vi "DO_init.vi"(0 "DOParameters":string[](array[string]), 1 "N_param":i32, 2 "N_moduls":i32, 5 "Parameters def":i32[][](array[numeric]), 7 "Names def":string[][](array[string]), 9 "KFM":string[](array[string]), 12 "conninfo":T1={"host"="localhost", "port"="5432", "client_encoding"="WIN1251", "dbname"="data", "user"="postgres", "password"=""}, 13 "DOParamTable":string="fdo_3") -> (4 "DO out":T2, 15 "error":errorcluster)   [LabVIEW 2019, in "Inputs.lvlib"]
uses:
  Inputs.lvlib
  Ctl/DO.ctl
  Ctl/Parameter State.ctl
  Database/ctl/Coninfo.ctl
  Database/PostgreSQL.lvlib
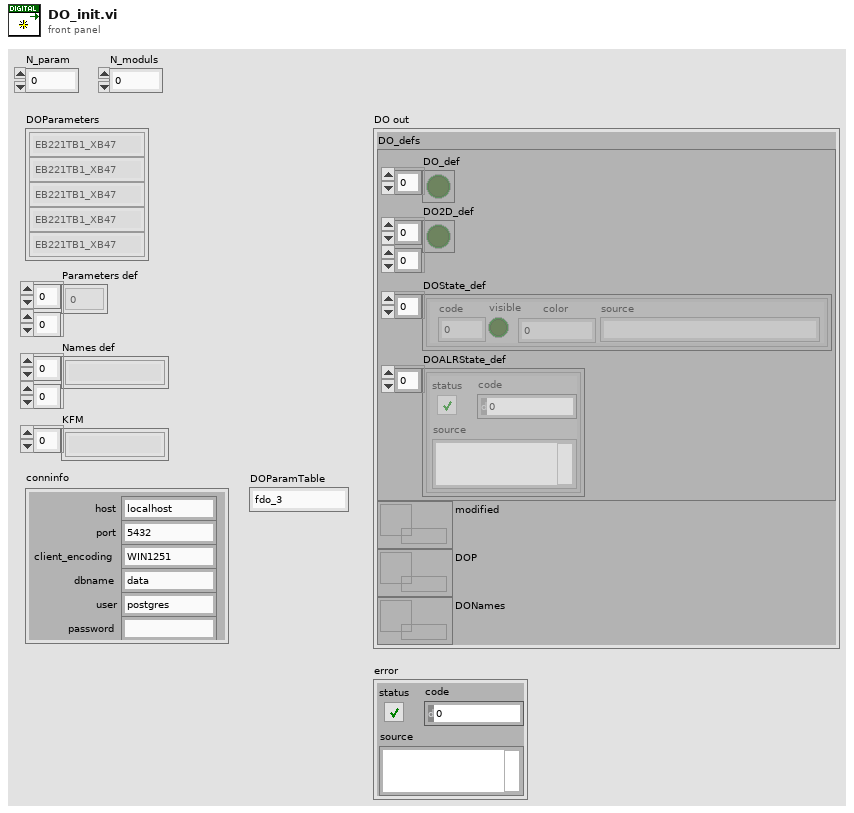
[diagram p1: front panel]
types:
  T1 = typedef "PostgreSQL.lvlib/Coninfo.ctl" = cluster{"host":string, "port":string, "client_encoding":string, "dbname":string, "user":string, "password":string}
  T2 = typedef "Inputs.lvlib/DO.ctl" = cluster{"DO_defs":cluster{"DO_def":bool[], "DO2D_def":bool[][], "DOState_def":T3[], "DOALRState_def":errorcluster[]}, "modified":refnum<data-value>, "DOP":refnum<data-value>, "DONames":refnum<data-value>}
  T3 = typedef "Inputs.lvlib/Parameter State.ctl" = cluster{"code":i32, "visible":bool, "color":u32, "source":string}
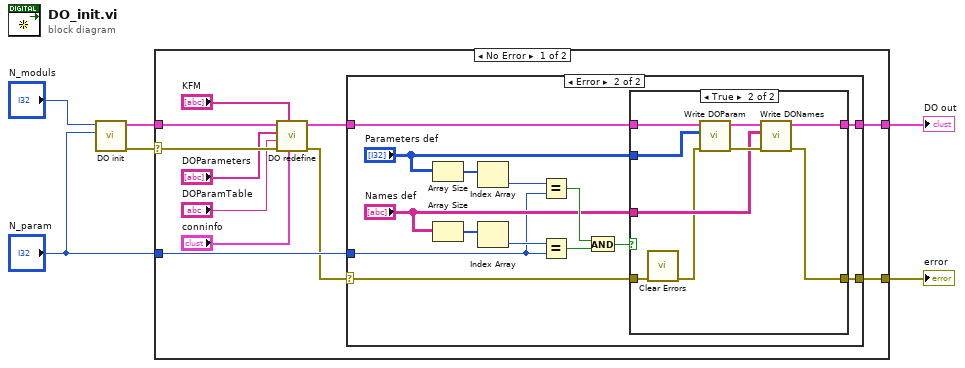
[diagram p0: block diagram]
diagram:
  n1 = call "DO init.vi"("N_param"="N_param", "N_moduls"="N_moduls") -> ("error"=w3:errorcluster, "DO"=w4:T2)  [unwired: 8 in]
  n2 = case shown="No Error" w3 {
    selector: w3 -> [w14 w46]
    tunnel: "N_param" -> [w16 _]
    tunnel: [w17 w46] -> w6
    tunnel: w4 -> [w13 w45]
    tunnel: [w15 w45] -> w2
    frame No Error {
      n3 = call "DO redefine.vi"("conninfo"="conninfo", "KFM"="KFM", "error in (no error)"=w14, "DOParamTable"="DOParamTable", "DOParameters"="DOParameters", "DO in"=w13) -> ("error"=w11:errorcluster, "DO out"=w12:T2)  [unwired: 4 in]
      n4 = case shown="Error" w11 {
        selector: w11 -> [w19 w24]
        tunnel: [w19 w25] -> w17
        tunnel: w16 -> [_ w26]
        tunnel: w12 -> [w18 w21]
        tunnel: [w18 w20] -> w15
        frame No Error {
        }
        frame Error {
          n5 = Array Size(array="Parameters def") -> (size(s)=w28:i32[])
          n6 = Array Size(array="Names def") -> (size(s)=w29:i32[])
          n7 = Index Array(array=w28) -> (element=w30:i32)  [unwired: 1 in]
          n8 = Index Array(array=w29) -> (element=w31:i32)  [unwired: 1 in]
          n9 = Equal?(x=w30, y=w26) -> (x = y?=w32:bool)
          n10 = Equal?(x=w31, y=w26) -> (x = y?=w33:bool)
          n11 = And(x=w32, y=w33) -> (x .and. y?=w22:bool)
          n12 = case shown="True" w22 {
            tunnel: "Parameters def" -> [_ w37]
            tunnel: "Names def" -> [_ w39]
            tunnel: [w34 w41] -> w25
            tunnel: w24 -> [w34 w38]
            tunnel: w21 -> [w35 w42]
            tunnel: [w35 w40] -> w20
            frame False {
            }
            frame True {
              n13 = call <vilib>:"Clear Errors.vi"("error in (no error)"=w38) -> ("error out"=w36:errorcluster)  [unwired: 5 in, 1 out]
              n14 = call "Write DOParam.vi"("error in (no error)"=w36, "DOParam"=w37, "DO in"=w42) -> ("error out"=w43:errorcluster, "DO out"=w44:T2)  [unwired: 7 in]
              n15 = call "Write DONames.vi"("error in (no error)"=w43, "DONames"=w39, "DO in"=w44) -> ("error out"=w41:errorcluster, "DO out"=w40:T2)  [unwired: 7 in]
            }
          }
        }
      }
    }
    frame Error {
    }
  }
  "DO out" <- w2
  "error" <- w6
